vi "RunTest.vi"(8 "error in (no error)":errorcluster, 11 "Prueba08 in":refnum<class "Prueba08.lvclass">) -> (0 "error out":errorcluster, 2 "resultado":string, 3 "Prueba08 out":refnum<class "Prueba08.lvclass">)   [LabVIEW 2019, in "Prueba08.lvclass"]
uses:
  Prueba08.lvclass
  Prueba04/Control/Slide.ctl
  MessageP08.ctl
  Controles/EstadosP08.ctl
  Prueba08.lvclass/Prueba08.ctl
  ClusterGEN.ctl
  <vilib>/Utility/error.llb/DialogType.ctl
  QMH/Message Queue/Enqueue Message (Single).vi
  <vilib>/Utility/error.llb/Error Cluster From Error Code.vi
  <vilib>/ErrorRing/Error Ring.xnode
  <vilib>/Utility/miscctls.llb/LVRowAndColumnTypeDef.ctl
  Prueba/Prueba.lvclass
  Prueba04/Prueba04.lvclass
  QMH/User Event - Stop/User Event - Stop.lvlib
  QMH/Message Queue/Message Queue.lvlib
panel:
  out "Leq":bool
  out "data":string
  out "fila_tabla":i32
  out "ms":dbl
  out "ms":string[](array[string])
  out "max value":dbl
  out "tablaTipoPondTemp":string[](array[string])
  out "tablaNivelMaxRef":string[](array[string])
  out "Pict Ring 2":u16(ring)
  out "Pict Ring 3":u16(ring)
  out "cumple_no_cumple":bool
  out "Vref":dbl
  in  "Tab":enum32{"Page 1", "Page 2"}(tab)
  out "NivelRMSensayo":dbl=95.0
  out "frecuencia1":dbl=140.0
  out "rangoRef":string
  in  "guardar_Vref":bool
  in  "generar1":bool
  in  "AjusteAmp":T1=50.0 caption="Ajuste de amplitud [mV]" scale=0.0..5000.0
  out "voltaje1":dbl format="%.1f"
  out "frecuencia1":dbl format="%.1f"
  in  "seguir":bool
  in  "guardarParamLEQ":bool caption="PruebaSup"
  in  "Tm":i32=60 min=60
  in  "N":i32=1 min=1 max=9
  in  "TablaTempotal":string[][](table)
  in  "cb_ponderacionTemp":string(combo)="0"
  in  "genera2":bool caption="PruebaSup"
  out "Tabla":string[][](table)
  in  "salir":bool
  out "cumple":bool
  out "no_cumple":bool
  out "voltaje2":dbl format="%#.1f"
  out "frecuencia2":dbl format="%#.1f"
  # "Elección Señal de Referencia\nsegún marca y modelo de sonómetro"
  # "Nivel RMS para Ensayo"
  # "Rango Referencia"
  # "Frecuencia"
  # "Monitoreo"
  # "Frecuencia"
  # "Hz"
  # "Voltaje"
  # "mV"
  # "8. Respuesta a trenes de ondas. IEC 61672-3: 2006 Cláusula 16"
  # "Tabla Resultados"
  # "Ingrese mediciones\naquí"
  # "Ingrese parámetros"
  # "Seleccione Tone Burst"
  # "N"
  # "Tm"
  # "Solo el máximo valor se \nregistrará en la tabla de Resultados"
  # "Cumple"
  # "No Cumple"
  # "8. Respuesta a trenes de ondas. IEC 61672-3: 2006 Cláusula 16"
  # "Monitoreo"
  # "Nivel RMS para Ensayo"
  # "dB"
  # "Voltaje"
  # "mV"
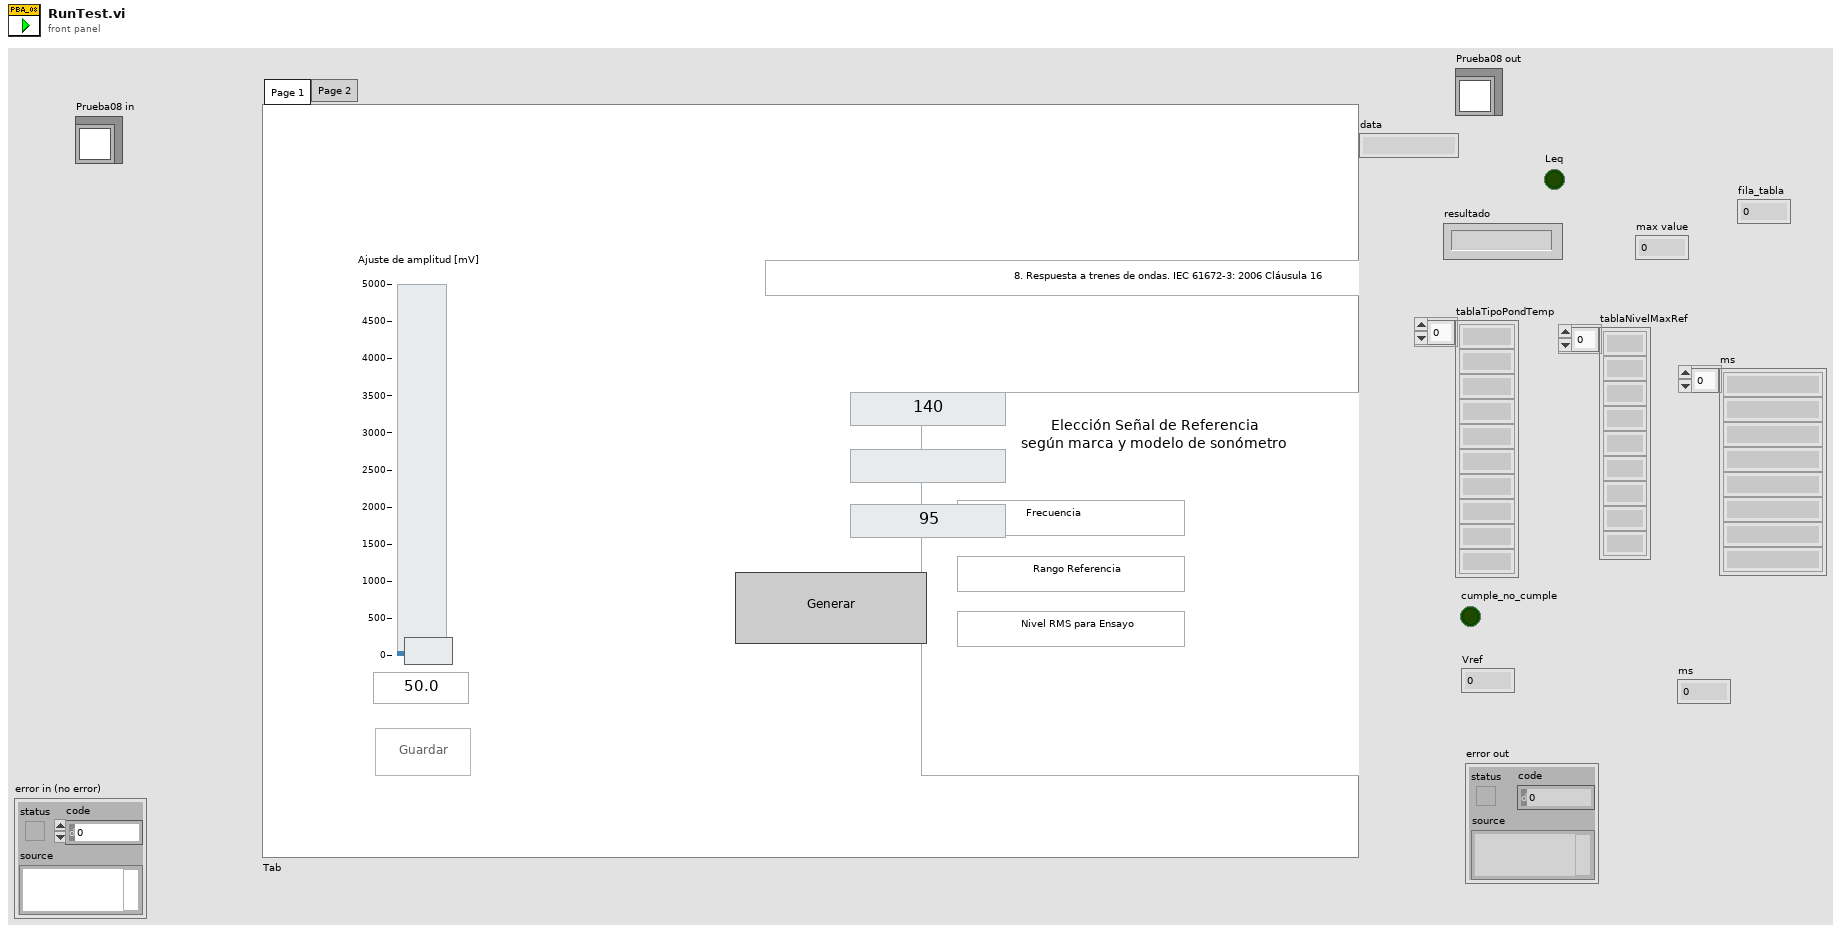
[diagram p1: front panel]
types:
  T1 = typedef "Prueba04.lvclass/Slide.ctl" = dbl
  T2 = typedef "LVRowAndColumnTypeDef.ctl" = cluster{"Row":i32, "Column":i32}
  T3 = typedef "Message Queue.lvlib/All Message Queues.ctl" = cluster{"MHL":refnum<queue>, "Inst_CNT90":refnum<queue>, "Inst_DS360":refnum<queue>, "Inst_Keithley2002":refnum<queue>, "Inst_DAQ":refnum<queue>, "BD":refnum<queue>, "Pistofono":refnum<queue>, "Nexus":refnum<queue>}
  T4 = enum32{"Page 1", "Page 2", "Page 3", "Page 4", "Page 5", "Page 6", "Page 7"}
  T5 = typedef "Prueba08.lvclass/ClusterGEN.ctl" = cluster{"frec":dbl, "amp":dbl, "ms_burst":dbl}
  T6 = enum8{"Enabled", "Disabled", "Disabled and Grayed Out"}
  T7 = cluster{"ControlName":string, "ControlReference":refnum<vi>}[]
  T8 = typedef "Prueba08.lvclass/MessageP08.ctl" = cluster{"Estados":T9, "Data":variant}
  T9 = typedef "Prueba08.lvclass/EstadosP08.ctl" = enum16{"Error", "DetieneInstrumentos", "InicializarInstrumentos", "inicio", "configuraTabla", "FrecAmp1", "FrecAmp2", "nivelMaxRef", "iniciarGEN", "iniciarGEN_burst", "detenerGEN", "llenaTablaTemporal", "guardaVref", "monitoreo", "ingresaMediciones", "guardaMediciones", "cumplimiento", "listo_evaluar", "evaluar", "LeerArchivoConfiguracion", "final", "salir"}
  T10 = typedef "DialogType.ctl" = u16
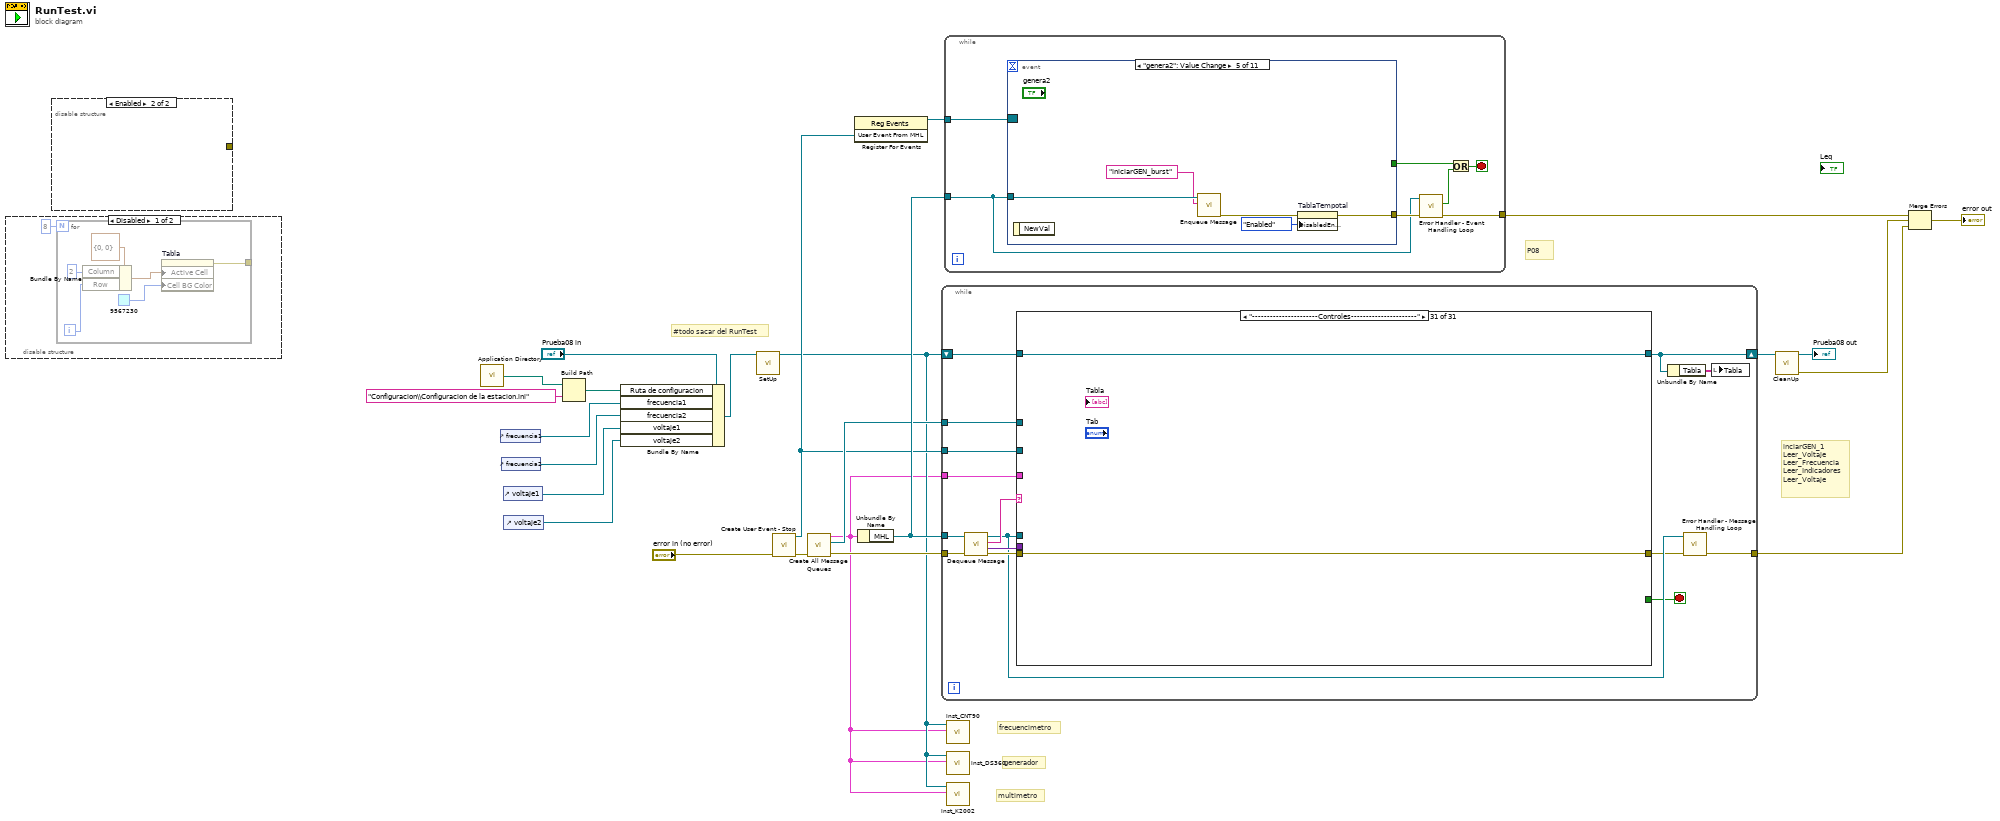
[diagram p0: block diagram]
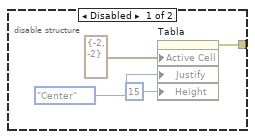
[diagram p3: hidden frame]
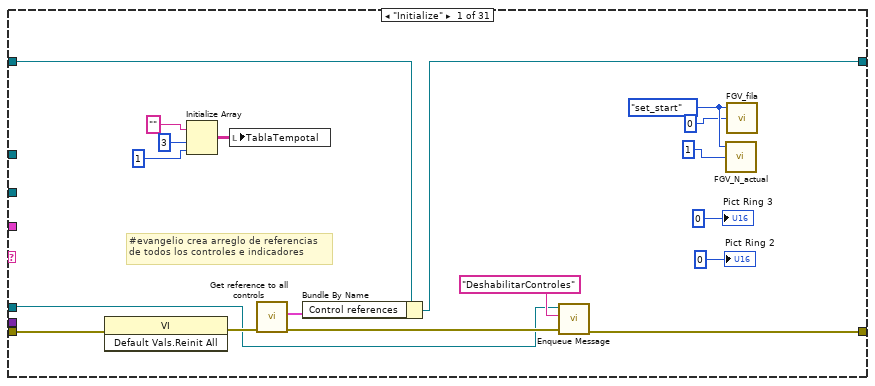
[diagram p4: hidden frame]
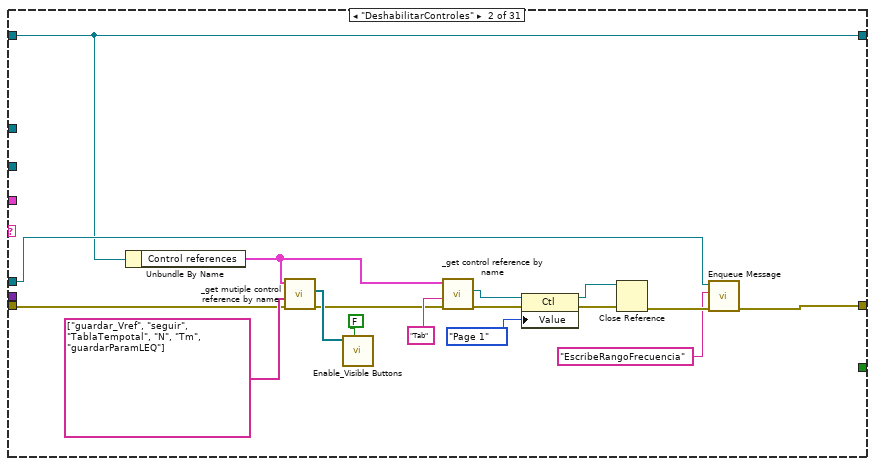
[diagram p5: hidden frame]
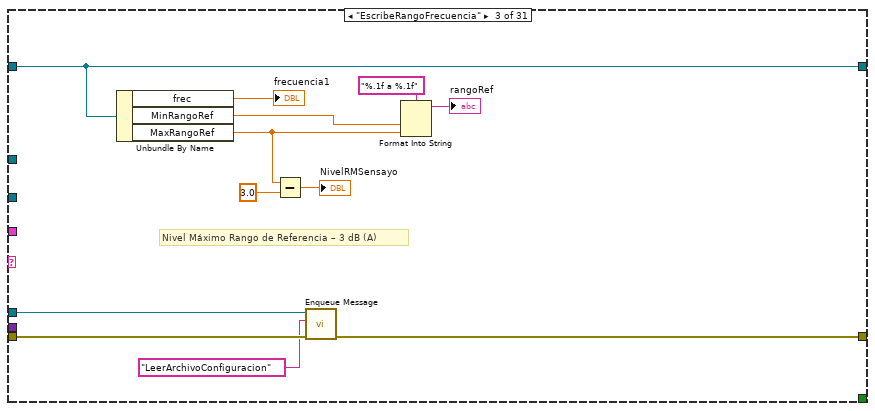
[diagram p6: hidden frame]
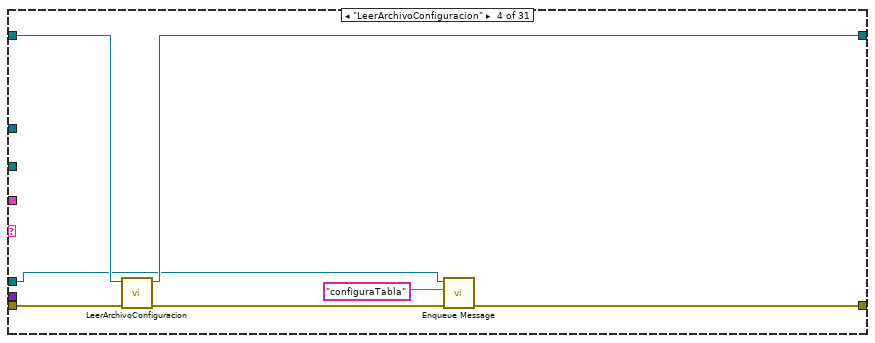
[diagram p7: hidden frame]
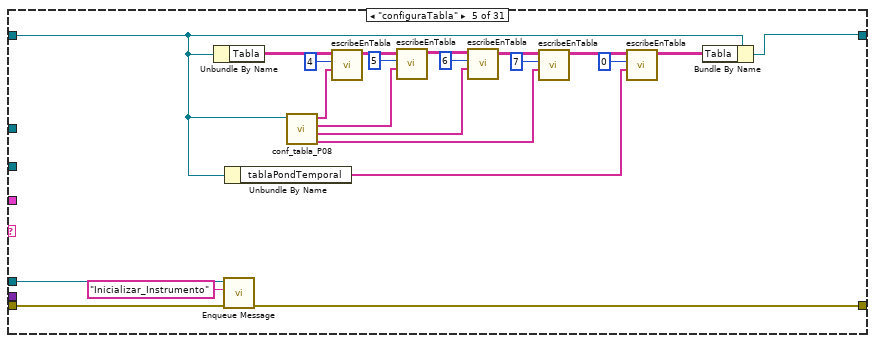
[diagram p8: hidden frame]
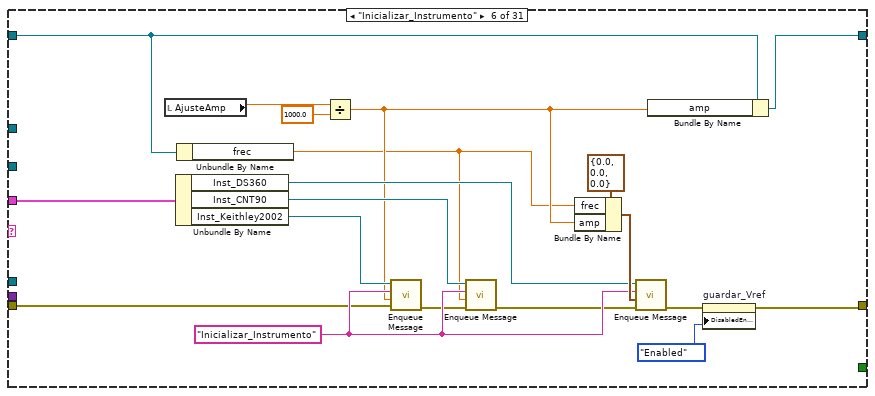
[diagram p9: hidden frame]
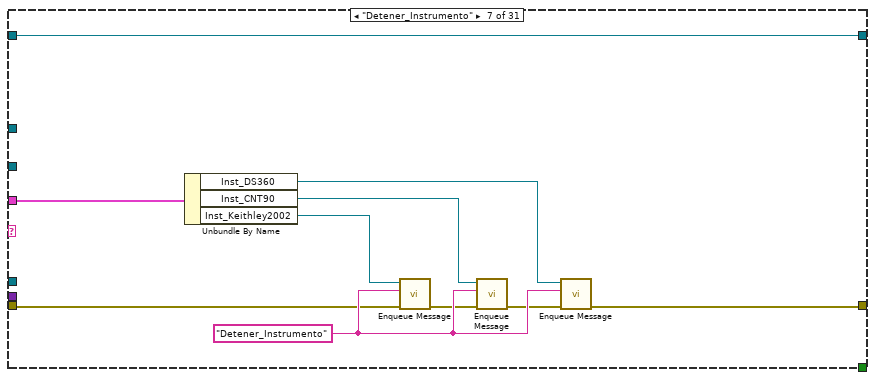
[diagram p10: hidden frame]
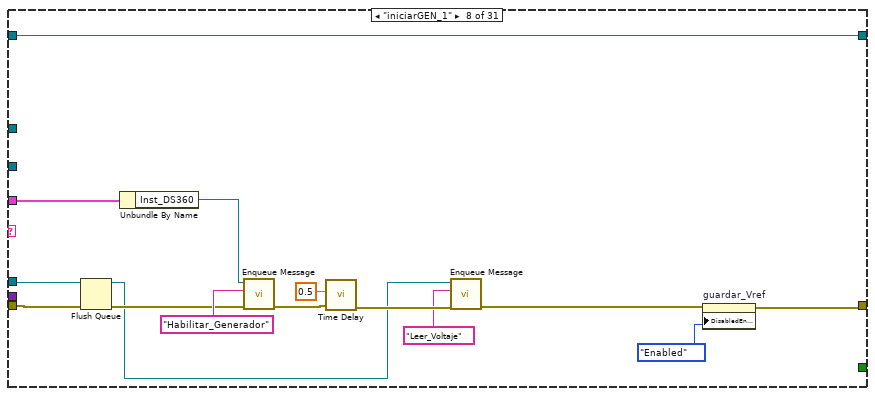
[diagram p11: hidden frame]
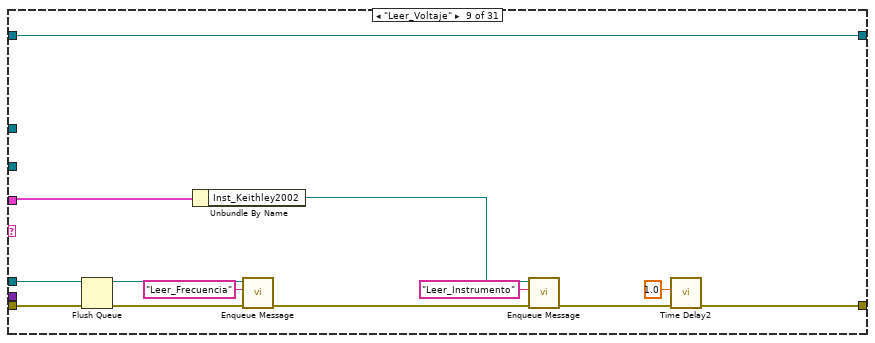
[diagram p12: hidden frame]
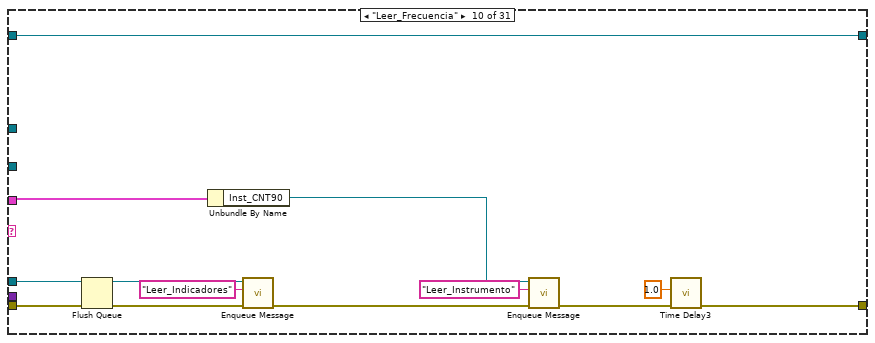
[diagram p13: hidden frame]
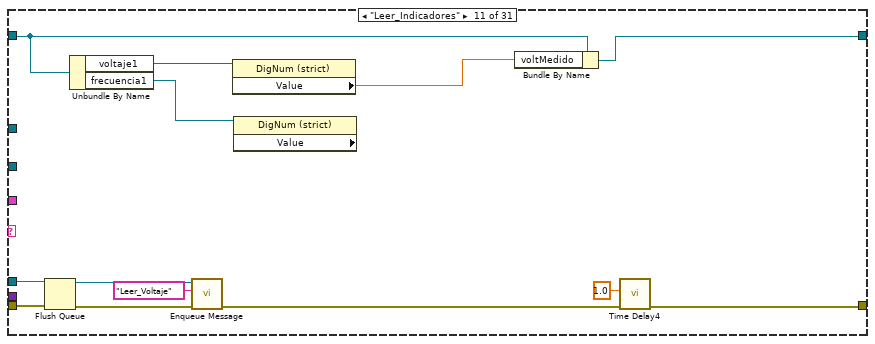
[diagram p14: hidden frame]
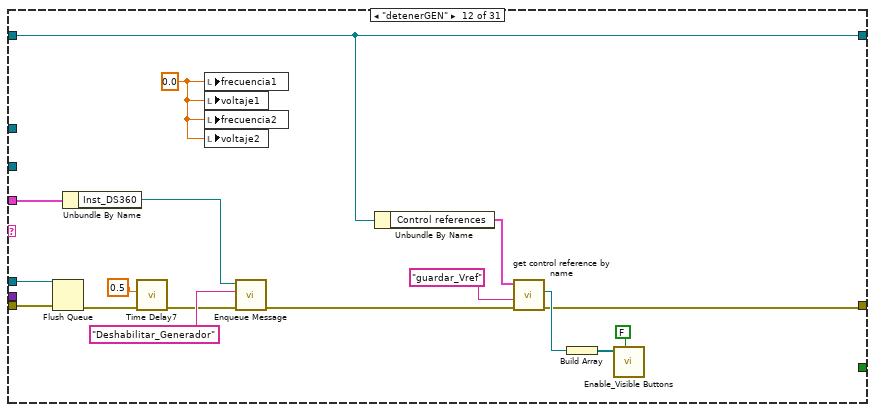
[diagram p15: hidden frame]
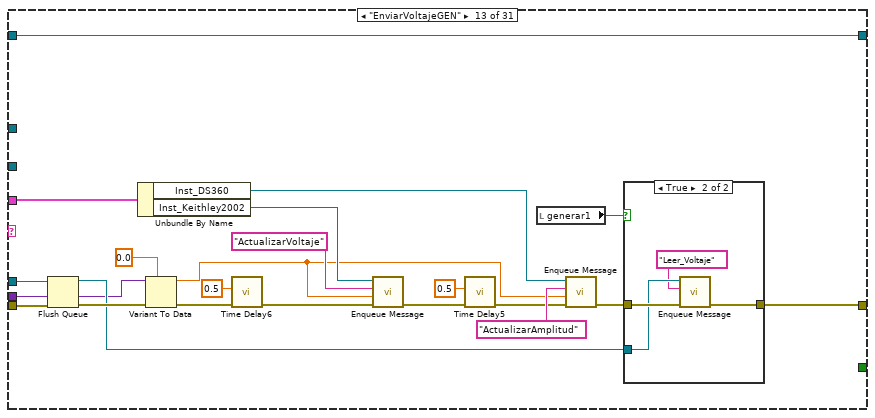
[diagram p16: hidden frame]
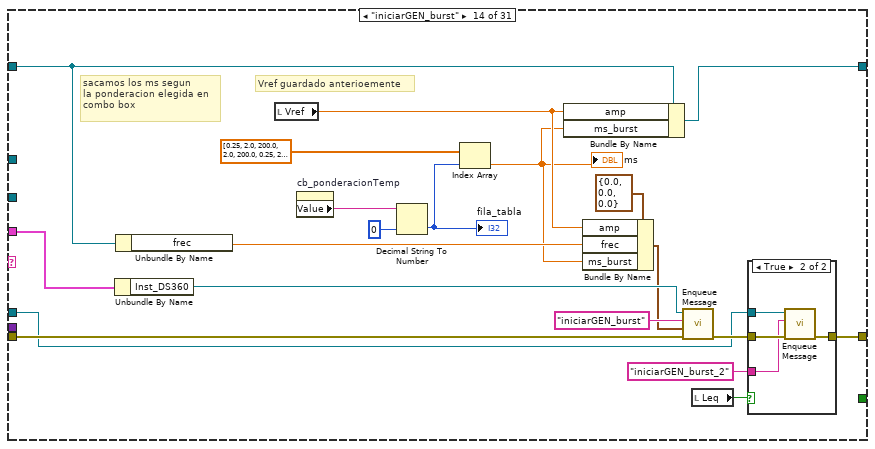
[diagram p18: hidden frame]
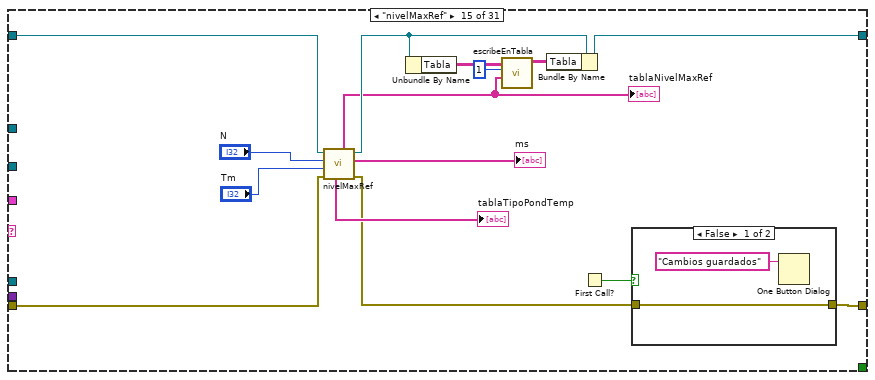
[diagram p20: hidden frame]
diagram:
  # "inciarGEN_1\nLeer_Voltaje\nLeer_Frecuencia\nLeer_Indicadores\nLeer_Voltaje"
  # "P08"
  # "multimetro"
  # "generador"
  # "frecuencimetro"
  # "#todo sacar del RunTest"
  n1 = disable-structure shown="Disabled" {
    frame Disabled {
      n2 = for {
        N: 8 -> [_]
        tunnel: [w27] -> _
        i -> [w26]
        n3 = Bundle By Name(cluster=T2 {"Row"=0, "Column"=0} ("Active Cell:Active Cell"), "Column"=2, "Row"=w26) -> (w29:T2)
        n4 = property on="Tabla" class="Tbl (strict)"("Active Cell"=w29, "Cell BG Color"=u32 9567230) -> (error out=w27:errorcluster)  [unwired: 2 in, 1 out]
      }
    }
    frame Enabled {
    }
  }
  n5 = disable-structure shown="Enabled" {
    disable-tunnel: [w34 _] -> _
    frame Disabled {
      n6 = property on="Tabla" class="Tbl (strict)"("Active Cell"=T2 {"Row"=-2, "Column"=-2} ("Active Cell:Active Cell"), "Justify"=enum16{"Left", "Center", "Right"}."Center" ("Active Cell:Cell Justification"), "Height"=u32 15 ("Active Cell:Cell Font:Size")) -> (error out=w34:errorcluster)  [unwired: 2 in, 1 out]
    }
    frame Enabled {
    }
  }
  n7 = call <vilib>:"Application Directory.vi"() -> ("Application Directory"=w19:path)
  n8 = control-ref of="frecuencia1"() -> (w8:refnum<vi>)
  n9 = control-ref of="frecuencia2"() -> (w7:refnum<vi>)
  n10 = control-ref of="voltaje1"() -> (w6:refnum<vi>)
  n11 = control-ref of="voltaje2"() -> (w5:refnum<vi>)
  n12 = Build Path(base path=w19, name or relative path="Configuracion\\Configuracion de la estacion.ini") -> (appended path=w18:path)
  n13 = Bundle By Name(cluster="Prueba08 in", "Ruta de configuracion"=w18, "frecuencia1"=w8, "frecuencia2"=w7, "voltaje1"=w6, "voltaje2"=w5) -> (w21:refnum<class "Prueba08.lvclass">)
  n14 = call-dynamic "SetUp.vi"("Prueba08 in"=w21) -> ("Prueba08 out"=w10:refnum<class "Prueba08.lvclass">)  [unwired: 9 in, 1 out]
  n15 = call "Create User Event - Stop.vi"("error in (no error)"="error in (no error)") -> ("error out"=w17:errorcluster, "User Event From MHL"=w12:refnum<user-event>)  [unwired: 9 in]
  n16 = call "Create All Message Queues.vi"("error in (no error)"=w17) -> ("error out"=w14:errorcluster, "PL Queues Array"=w13:refnum<queue>[], "All Message Queues out"=w9:T3)  [unwired: 8 in]
  n17 = register-events(w12) -> (reference out=w11:refnum<event-registration>)  [unwired: 2 in, 1 out]
  n18 = Unbundle By Name(w9) -> ("MHL"=w15:refnum<queue>)
  n19 = while {
    tunnel: w15 -> [w47]
    tunnel: w14 -> [w46]
    tunnel: [w40] -> w2
    shift-right: [w48] -> w4
    shift-left: w10 -> [w49]
    tunnel: w9 -> [w39]
    tunnel: w13 -> [w38]
    tunnel: w12 -> [w37]
    stop <- w36 stop-if-true
    n20 = call "Dequeue Message.vi"("error in (no error)"=w46, "Message Queue"=w47) -> ("error out"=w45:errorcluster, "Message Data"=w44:variant, "Message"=w43:string, "dup Message Queue"=w42:refnum<queue>)  [unwired: 6 in]
    n21 = case shown="\"----------------------Controles----------------------\"" w43 {
      selector: w43 -> [_ _ _ _ _ _ _ _ _ _ _ _ _ _ _ _ _ _ _ _ _ _ _ _ _ _ _ w474 _ w504 _]
      tunnel: w44 -> [_ _ _ _ _ _ _ _ _ _ _ _ w229 _ _ w305 w333 _ _ _ _ _ _ w434 w445 _ w468 _ _ _ _]
      tunnel: w45 -> [w64 w72 w89 w104 w120 w133 w148 w169 w174 w187 w204 w218 w231 w273 w292 w306 w340 w355 w372 w381 w397 w403 w415 w437 w448 w450 w469 w478 w489 _ w513]
      tunnel: [w62 w69 w86 w98 w107 w129 w147 w166 w171 w184 w200 w220 w228 w257 w280 w299 w339 w356 w370 w380 w395 w403 w419 w431 w443 w449 w463 w471 w487 w503 w513] -> w41
      tunnel: w42 -> [w63 w71 w88 w100 w106 _ _ w168 w173 w186 w203 w217 w230 w256 _ _ w337 w353 w369 w379 w396 _ w420 _ _ _ w462 w477 w488 _ _]
      tunnel: [w53 w70 w97 w103 w117 w145 w155 w165 w183 w196 w201 w216 w248 w272 w287 w302 w334 w364 w368 w376 w393 w404 w422 w435 w446 w453 w470 w473 w494 w505 w514] -> w48
      tunnel: w49 -> [w54 w70 w97 w102 w109 w128 w155 w165 w183 w196 w202 w216 w248 w261 w293 w302 w334 w365 w367 w376 w393 w404 w422 w436 w447 w453 w470 w473 w494 w505 w514]
      tunnel: w39 -> [_ _ _ _ _ w132 w146 w167 w172 w185 _ w219 w232 w267 _ _ _ _ _ _ _ _ _ _ _ _ _ _ _ _ _]
      tunnel: w38 -> [_ _ _ _ _ _ _ _ _ _ _ _ _ _ _ _ _ _ _ _ _ _ _ _ _ _ _ w476 _ _ _]
      tunnel: w37 -> [_ _ _ _ _ _ _ _ _ _ _ _ _ _ _ _ _ _ _ _ _ _ _ _ _ _ _ w475 _ _ _]
      tunnel: [_ _ _ _ _ _ _ _ _ _ _ _ _ _ _ _ _ _ _ _ _ _ _ _ _ _ _ w472 _ _ _] -> w36
      frame "Initialize" {
        w56 = enum16{"increment", "set_start", "get"}."set_start" ("action")
        # "#evangelio crea arreglo de referencias\nde todos los controles e indicadores"
        n22 = invoke class="VI" method="Default Vals.Reinit All"(error in=w64) -> (error out=w67:errorcluster)  [unwired: 2 in, 2 out]
        n23 = Initialize Array("", 3 ("dimension size"), 1 ("dimension size")) -> (w61:string[][])
        n24 = local write "TablaTempotal"(w61) -> ()
        n25 = call "Get reference to all controls.vi"("error in (no error)"=w67) -> ("error out"=w65:errorcluster, "Control references"=w66:T7)  [unwired: 5 in]
        n26 = Bundle By Name(cluster=w54, "Control references"=w66) -> (w53:refnum<class "Prueba08.lvclass">)
        n27 = call-poly "Enqueue Message.vi"("error in (no error)"=w65, "Message"="DeshabilitarControles", "Message Queue"=w63) -> ("error out"=w62:errorcluster)  [unwired: 7 in, 1 out]
        n28 = call "FGV_N_actual.vi"("N_actual in"=1 ("fila_inicial"), "action"=w56) -> ()  [unwired: 2 in, 2 out]
        n29 = call "FGV_fila.vi"("fila_inicial"=0, "action"=w56) -> ()  [unwired: 2 in, 2 out]
        "Pict Ring 2" <- u16 0 ("Pict Ring 2")
        "Pict Ring 3" <- u16 0 ("Pict Ring 3")
      }
      frame "DeshabilitarControles" {
        n30 = Unbundle By Name(w70) -> ("Control references"=w81:T7)
        n31 = call "_get mutiple control reference by name.vi"("error in (no error)"=w72, "Control names"=string[] ["guardar_Vref", "seguir", "TablaTempotal", "N", "Tm", "guardarParamLEQ"], "Control references"=w81) -> ("error out"=w78:errorcluster, "References"=w79:refnum<vi>[])  [unwired: 3 in]
        n32 = call "Enable_Visible Buttons.vi"("Enable? (T)"=FALSE, "Controls Ref Array"=w79) -> ()  [unwired: 10 in]
        n33 = call "_get control reference by name.vi"("error in (no error)"=w78, "Control name"="Tab" ("Message"), "Control references"=w81) -> ("error out"=w85:errorcluster, "Ctl Refnum"=w83:refnum<vi>)  [unwired: 3 in]
        n34 = property class="Ctl"(reference=w83, error in=w85, "Value"=T4."Page 1" ("Tab_Prueba04")) -> (reference out=w74:refnum<vi>, error out=w76:errorcluster)
        n35 = Close Reference(reference=w74, error in (no error)=w76) -> (error out=w75:errorcluster)
        n36 = call-poly "Enqueue Message.vi"("error in (no error)"=w75, "Message"="EscribeRangoFrecuencia", "Message Queue"=w71) -> ("error out"=w69:errorcluster)  [unwired: 7 in, 1 out]
      }
      frame "EscribeRangoFrecuencia" {
        # "Nivel Máximo Rango de Referencia – 3 dB (A)"
        n37 = Unbundle By Name(w97) -> ("frec"=→"frecuencia1":dbl, "MinRangoRef"=w93:dbl, "MaxRangoRef"=w92:dbl)
        n38 = Subtract(x=w92, y=3.0) -> (x-y=→"NivelRMSensayo":dbl)
        n39 = call-poly "Enqueue Message.vi"("error in (no error)"=w89, "Message"="LeerArchivoConfiguracion", "Message Queue"=w88) -> ("error out"=w86:errorcluster)  [unwired: 7 in, 1 out]
        n40 = Format Into String(format string="%.1f a %.1f", w93, w92) -> (resulting string=→"rangoRef":string)  [unwired: 2 in, 1 out]
      }
      frame "LeerArchivoConfiguracion" {
        n41 = call "LeerArchivoConfiguracion.vi"("error in"=w104, "Prueba31 in"=w102) -> ("error out"=w101:errorcluster, "Prueba31 out"=w103:refnum<class "Prueba08.lvclass">)  [unwired: 8 in]
        n42 = call-poly "Enqueue Message.vi"("error in (no error)"=w101, "Message"="configuraTabla", "Message Queue"=w100) -> ("error out"=w98:errorcluster)  [unwired: 7 in, 1 out]
      }
      frame "configuraTabla" {
        n43 = Unbundle By Name(w109) -> ("Tabla"=w116:string[][])
        n44 = call-poly "Enqueue Message.vi"("error in (no error)"=w120, "Message"="Inicializar_Instrumento", "Message Queue"=w106) -> ("error out"=w107:errorcluster)  [unwired: 7 in, 1 out]
        n45 = Unbundle By Name(w109) -> ("tablaPondTemporal"=w108:string[])
        n46 = call "conf_tabla_P08.vi"("Prueba07 out"=w109) -> ("cumplimiento"=w112:string[], "Tol -"=w113:string[], "Tol +"=w114:string[], "incertidumbre"=w115:string[])  [unwired: 7 in]
        n47 = call "escribeEnTabla.vi"("parametros"=w115, "col"=4, "tabla in"=w116) -> ("tabla out"=w126:string[][])  [unwired: 8 in]
        n48 = call "escribeEnTabla.vi"("parametros"=w114, "col"=5, "tabla in"=w126) -> ("tabla out"=w125:string[][])  [unwired: 8 in]
        n49 = call "escribeEnTabla.vi"("parametros"=w113, "col"=6, "tabla in"=w125) -> ("tabla out"=w121:string[][])  [unwired: 8 in]
        n50 = call "escribeEnTabla.vi"("parametros"=w112, "col"=7, "tabla in"=w121) -> ("tabla out"=w119:string[][])  [unwired: 8 in]
        n51 = call "escribeEnTabla.vi"("parametros"=w108, "col"=0, "tabla in"=w119) -> ("tabla out"=w111:string[][])  [unwired: 8 in]
        n52 = Bundle By Name(cluster=w109, "Tabla"=w111) -> (w117:refnum<class "Prueba08.lvclass">)
      }
      frame "Inicializar_Instrumento" {
        w140 = "Inicializar_Instrumento" ("Message")
        n53 = local read "AjusteAmp"() -> (w144:T1)
        n54 = Unbundle By Name(w132) -> ("Inst_DS360"=w135:refnum<queue>, "Inst_CNT90"=w134:refnum<queue>, "Inst_Keithley2002"=w142:refnum<queue>)
        n55 = Unbundle By Name(w128) -> ("frec"=w127:dbl)
        n56 = Divide(x=w144, y=T1 1000.0) -> (x/y=w130:T1)
        n57 = call-poly "Enqueue Message.vi"("error in (no error)"=w133, "Message Data"=w130, "Message"=w140, "Message Queue"=w142) -> ("error out"=w139:errorcluster)  [unwired: 6 in, 1 out]
        n58 = call-poly "Enqueue Message.vi"("error in (no error)"=w139, "Message Data"=w127, "Message"=w140, "Message Queue"=w134) -> ("error out"=w138:errorcluster)  [unwired: 6 in, 1 out]
        n59 = Bundle By Name(cluster=T5 {"frec"=0.0, "amp"=0.0, "ms_burst"=0.0} ("clusterGEN"), "frec"=w127, "amp"=w130) -> (w141:T5)
        n60 = call-poly "Enqueue Message.vi"("error in (no error)"=w138, "Message Data"=w141, "Message"=w140, "Message Queue"=w135) -> ("error out"=w136:errorcluster)  [unwired: 6 in, 1 out]
        n61 = Bundle By Name(cluster=w128, "amp"=w130) -> (w145:refnum<class "Prueba08.lvclass">)
        n62 = property on="guardar_Vref" class="Bool"(error in=w136, "DisabledEnum"=T6."Enabled" ("Disabled")) -> (error out=w129:errorcluster)  [unwired: 1 in, 1 out]
      }
      frame "Detener_Instrumento" {
        w151 = "Detener_Instrumento" ("Message")
        n63 = Unbundle By Name(w146) -> ("Inst_DS360"=w154:refnum<queue>, "Inst_CNT90"=w153:refnum<queue>, "Inst_Keithley2002"=w152:refnum<queue>)
        n64 = call-poly "Enqueue Message.vi"("error in (no error)"=w148, "Message"=w151, "Message Queue"=w152) -> ("error out"=w150:errorcluster)  [unwired: 7 in, 1 out]
        n65 = call-poly "Enqueue Message.vi"("error in (no error)"=w150, "Message"=w151, "Message Queue"=w153) -> ("error out"=w149:errorcluster)  [unwired: 7 in, 1 out]
        n66 = call-poly "Enqueue Message.vi"("error in (no error)"=w149, "Message"=w151, "Message Queue"=w154) -> ("error out"=w147:errorcluster)  [unwired: 7 in, 1 out]
      }
      frame "iniciarGEN_1" {
        n67 = Flush Queue(queue=w168, error in (no error)=w169) -> (queue out=w156:refnum<queue>, error out=w159:errorcluster)  [unwired: 1 out]
        n68 = Unbundle By Name(w167) -> ("Inst_DS360"=w157:refnum<queue>)
        n69 = call-poly "Enqueue Message.vi"("error in (no error)"=w159, "Message"="Habilitar_Generador", "Message Queue"=w157) -> ("error out"=w162:errorcluster)  [unwired: 7 in, 1 out]
        n70 = call "Time Delay"("error in (no error)"=w162, "Delay Time (s)"=0.5) -> ("error out"=w161:errorcluster)  [unwired: 9 in]
        n71 = call-poly "Enqueue Message.vi"("error in (no error)"=w161, "Message"="Leer_Voltaje", "Message Queue"=w156) -> ("error out"=w158:errorcluster)  [unwired: 7 in, 1 out]
        n72 = property on="guardar_Vref" class="Bool"(error in=w158, "DisabledEnum"=T6."Enabled" ("Disabled")) -> (error out=w166:errorcluster)  [unwired: 1 in, 1 out]
      }
      frame "Leer_Voltaje" {
        n73 = Flush Queue(queue=w173, error in (no error)=w174) -> (queue out=w175:refnum<queue>, error out=w176:errorcluster)  [unwired: 1 out]
        n74 = Unbundle By Name(w172) -> ("Inst_Keithley2002"=w179:refnum<queue>)
        n75 = call-poly "Enqueue Message.vi"("error in (no error)"=w176, "Message"="Leer_Frecuencia", "Message Queue"=w175) -> ("error out"=w182:errorcluster)  [unwired: 7 in, 1 out]
        n76 = call-poly "Enqueue Message.vi"("error in (no error)"=w182, "Message"="Leer_Instrumento", "Message Queue"=w179) -> ("error out"=w180:errorcluster)  [unwired: 7 in, 1 out]
        n77 = call "Time Delay2"("error in (no error)"=w180, "Delay Time (s)"=1.0) -> ("error out"=w171:errorcluster)  [unwired: 9 in]
      }
      frame "Leer_Frecuencia" {
        n78 = Flush Queue(queue=w186, error in (no error)=w187) -> (queue out=w188:refnum<queue>, error out=w189:errorcluster)  [unwired: 1 out]
        n79 = Unbundle By Name(w185) -> ("Inst_CNT90"=w192:refnum<queue>)
        n80 = call-poly "Enqueue Message.vi"("error in (no error)"=w189, "Message"="Leer_Indicadores", "Message Queue"=w188) -> ("error out"=w195:errorcluster)  [unwired: 7 in, 1 out]
        n81 = call-poly "Enqueue Message.vi"("error in (no error)"=w195, "Message"="Leer_Instrumento", "Message Queue"=w192) -> ("error out"=w193:errorcluster)  [unwired: 7 in, 1 out]
        n82 = call "Time Delay3"("error in (no error)"=w193, "Delay Time (s)"=1.0) -> ("error out"=w184:errorcluster)  [unwired: 9 in]
      }
      frame "Leer_Indicadores" {
        n83 = Flush Queue(queue=w203, error in (no error)=w204) -> (queue out=w205:refnum<queue>, error out=w206:errorcluster)  [unwired: 1 out]
        n84 = Unbundle By Name(w202) -> ("voltaje1"=w199:refnum<vi>, "frecuencia1"=w198:refnum<vi>)
        n85 = call-poly "Enqueue Message.vi"("error in (no error)"=w206, "Message"="Leer_Voltaje", "Message Queue"=w205) -> ("error out"=w209:errorcluster)  [unwired: 7 in, 1 out]
        n86 = property class="DigNum (strict)"(reference=w199) -> ("Value"=w197:dbl)  [unwired: 1 in, 2 out]
        n87 = property class="DigNum (strict)" props=["Value"](reference=w198) -> ()  [unwired: 1 in, 3 out]
        n88 = Bundle By Name(cluster=w202, "voltMedido"=w197) -> (w201:refnum<class "Prueba08.lvclass">)
        n89 = call "Time Delay4"("error in (no error)"=w209, "Delay Time (s)"=1.0) -> ("error out"=w200:errorcluster)  [unwired: 9 in]
      }
      frame "detenerGEN" {
        w215 = 0.0 ("frecuencia1")
        n90 = Flush Queue(queue=w217, error in (no error)=w218) -> (error out=w212:errorcluster)  [unwired: 2 out]
        n91 = Unbundle By Name(w219) -> ("Inst_DS360"=w226:refnum<queue>)
        n92 = call "Time Delay7"("error in (no error)"=w212, "Delay Time (s)"=0.5) -> ("error out"=w211:errorcluster)  [unwired: 9 in]
        n93 = local write "frecuencia1"(w215) -> ()
        n94 = local write "voltaje1"(w215) -> ()
        n95 = local write "frecuencia2"(w215) -> ()
        n96 = local write "voltaje2"(w215) -> ()
        n97 = call-poly "Enqueue Message.vi"("error in (no error)"=w211, "Message"="Deshabilitar_Generador", "Message Queue"=w226) -> ("error out"=w210:errorcluster)  [unwired: 7 in, 1 out]
        n98 = Unbundle By Name(w216) -> ("Control references"=w221:T7)
        n99 = call-poly "get control reference by name.vi"("error in (no error)"=w210, "Control name"="guardar_Vref" ("String"), "Control references"=w221) -> ("error out"=w220:errorcluster, "Ctl Refnum"=w223:refnum<vi>)  [unwired: 3 in]
        n100 = Build Array(w223) -> (w222:refnum<vi>[])
        n101 = call "Enable_Visible Buttons.vi"("Enable? (T)"=FALSE, "Controls Ref Array"=w222) -> ()  [unwired: 10 in]
      }
      frame "EnviarVoltajeGEN" {
        n102 = Flush Queue(queue=w230, error in (no error)=w231) -> (queue out=w235:refnum<queue>, error out=w238:errorcluster)  [unwired: 1 out]
        n103 = Unbundle By Name(w232) -> ("Inst_DS360"=w242:refnum<queue>, "Inst_Keithley2002"=w247:refnum<queue>)
        n104 = Variant To Data(error in=w238, type=0.0, Variant=w229) -> (data=w240:dbl, error out=w245:errorcluster)
        n105 = call "Time Delay6"("error in (no error)"=w245, "Delay Time (s)"=0.5) -> ("error out"=w234:errorcluster)  [unwired: 9 in]
        n106 = call-poly "Enqueue Message.vi"("error in (no error)"=w234, "Message Data"=w240, "Message"="ActualizarVoltaje", "Message Queue"=w247) -> ("error out"=w243:errorcluster)  [unwired: 6 in, 1 out]
        n107 = call "Time Delay5"("error in (no error)"=w243, "Delay Time (s)"=0.5) -> ("error out"=w237:errorcluster)  [unwired: 9 in]
        n108 = local read "generar1"() -> (w227:bool)
        n109 = call-poly "Enqueue Message.vi"("error in (no error)"=w237, "Message Data"=w240, "Message"="ActualizarAmplitud", "Message Queue"=w242) -> ("error out"=w239:errorcluster)  [unwired: 6 in, 1 out]
        n110 = case shown="True" w227 {
          tunnel: w239 -> [w249 w253]
          tunnel: [w249 w252] -> w228
          tunnel: w235 -> [_ w251]
          frame False {
          }
          frame True {
            n111 = call-poly "Enqueue Message.vi"("error in (no error)"=w253, "Message"="Leer_Voltaje", "Message Queue"=w251) -> ("error out"=w252:errorcluster)  [unwired: 7 in, 1 out]
          }
        }
      }
      frame "iniciarGEN_burst" {
        # "sacamos los ms segun\nla ponderacion elegida en\ncombo box"
        # "Vref guardado anterioemente"
        n112 = Unbundle By Name(w267) -> ("Inst_DS360"=w266:refnum<queue>)
        n113 = Unbundle By Name(w261) -> ("frec"=w260:dbl)
        n114 = local read "Vref"() -> (w262:dbl)
        n115 = property on="cb_ponderacionTemp" class="CmbBox"() -> ("Value"=w270:string)  [unwired: 2 in, 2 out]
        n116 = Decimal String To Number(string=w270, default (0L)=0 ("default (0 I32)")) -> (number=w268:i32)  [unwired: 1 in, 1 out]
        "fila_tabla" <- w268
        n117 = Index Array(array=dbl[] [0.25, 2.0, 200.0, 2.0, 200.0, 0.25, 2.0, 200.0], index=w268) -> (element=w259:dbl)
        "ms" <- w259
        n118 = Bundle By Name(cluster=w261, "amp"=w262, "ms_burst"=w259) -> (w272:refnum<class "Prueba08.lvclass">)
        n119 = Bundle By Name(cluster=T5 {"frec"=0.0, "amp"=0.0, "ms_burst"=0.0} ("clusterGEN"), "amp"=w262, "frec"=w260, "ms_burst"=w259) -> (w263:T5)
        n120 = call-poly "Enqueue Message.vi"("error in (no error)"=w273, "Message Data"=w263, "Message"="iniciarGEN_burst", "Message Queue"=w266) -> ("error out"=w258:errorcluster)  [unwired: 6 in, 1 out]
        n121 = local read "Leq"() -> (w255:bool)
        n122 = case shown="True" w255 {
          tunnel: w258 -> [w274 w278]
          tunnel: [w274 w277] -> w257
          tunnel: w256 -> [_ w276]
          tunnel: "iniciarGEN_burst_2" ("Message") -> [_ w275]
          frame False {
          }
          frame True {
            n123 = call-poly "Enqueue Message.vi"("error in (no error)"=w278, "Message"=w275, "Message Queue"=w276) -> ("error out"=w277:errorcluster)  [unwired: 7 in, 1 out]
          }
        }
      }
      frame "nivelMaxRef" {
        n124 = call "nivelMaxRef.vi"("error in (no error)"=w292, "Tm"="Tm", "N"="N", "Prueba08 in"=w293) -> ("error out"=w281:errorcluster, "ms"=→"ms":string[], "Prueba08 out"=w291:refnum<class "Prueba08.lvclass">, "tablaNivelMaxRef"=w288:string[], "tablaTipoPondTemp"=→"tablaTipoPondTemp":string[])  [unwired: 2 in, 1 out]
        "tablaNivelMaxRef" <- w288
        n125 = Unbundle By Name(w291) -> ("Tabla"=w290:string[][])
        n126 = call "escribeEnTabla.vi"("parametros"=w288, "col"=1, "tabla in"=w290) -> ("tabla out"=w286:string[][])  [unwired: 8 in]
        n127 = Bundle By Name(cluster=w291, "Tabla"=w286) -> (w287:refnum<class "Prueba08.lvclass">)
        n128 = First Call?() -> (First Call?: T/F=w279:bool)
        n129 = case shown="False" w279 {
          tunnel: w281 -> [w294 w296]
          tunnel: [w294 w296] -> w280
          frame False {
            n130 = One Button Dialog(message="Cambios guardados") -> ()  [unwired: 1 in, 1 out]
          }
          frame True {
          }
        }
      }
      frame "TipoPonderacionTemporal" {
        n131 = Variant To Data(error in=w306, type="", Variant=w305) -> (data=w303:string, error out=w300:errorcluster)
        "data" <- w303
        n132 = Unbundle By Name(w302) -> ("Control references"=w301:T7)
        n133 = case shown="\"5\", \"6\", \"7\"" w303 {
          tunnel: w301 -> [w310 w317]
          tunnel: w300 -> [w309 w316]
          tunnel: [w311 w318] -> w299
          tunnel: string[] ["N", "Tm", "guardarParamLEQ"] ("String") -> [w308 w315]
          tunnel: [TRUE FALSE] -> w297
          frame "5", "6", "7" {
            # "Opcion Leq"
            n134 = call-poly "get control reference by name.vi"("error in (no error)"=w309, "Control names"=w308, "Control references"=w310) -> ("error out"=w311:errorcluster, "References"=w312:refnum<vi>[])  [unwired: 3 in]
            n135 = call "Enable_Visible Buttons.vi"("Enable? (T)"=TRUE, "Controls Ref Array"=w312) -> ()  [unwired: 10 in]
          }
          frame Default {
            # "No es Leq"
            n136 = call-poly "get control reference by name.vi"("error in (no error)"=w316, "Control names"=w315, "Control references"=w317) -> ("error out"=w318:errorcluster, "References"=w319:refnum<vi>[])  [unwired: 3 in]
            n137 = call "Enable_Visible Buttons.vi"("Enable? (T)"=FALSE, "Controls Ref Array"=w319) -> ()  [unwired: 10 in]
          }
        }
        n138 = local write "Leq"(w297) -> ()
      }
      frame "llenaTablaTemporal" {
        n139 = Flush Queue(queue=w337, error in (no error)=w340) -> (queue out=w336:refnum<queue>, error out=w338:errorcluster)  [unwired: 1 out]
        n140 = Variant To Data(error in=w338, type=string[][] [] ("NewVal"), Variant=w333) -> (data=w331:string[][], error out=w330:errorcluster)
        n141 = control-ref of="TablaTempotal"() -> (w332:refnum<vi>)
        n142 = call "llenaTablaTemporal.vi"("Tbl Refnum"=w332, "New Value"=w331, "error out"=w330) -> ("max value"=w321:dbl, "error in (no error)"=w329:errorcluster)  [unwired: 6 in]
        "max value" <- w321
        n143 = call "FGV_fila.vi"("error in (no error)"=w329, "action"=enum16{"increment", "set_start", "get"}."increment") -> ("error out"=w328:errorcluster)  [unwired: 2 in, 1 out]
        n144 = call "FGV_fila.vi"("error in (no error)"=w328, "action"=enum16{"increment", "set_start", "get"}."get") -> ("error out"=w326:errorcluster, "fila out"=w324:i32)  [unwired: 2 in]
        n145 = Greater?(x=w324, y=2) -> (0:w322:bool)
        n146 = case shown="True" w322 {
          tunnel: [w341 w350] -> w339
          tunnel: w336 -> [_ w349]
          tunnel: w326 -> [w341 w348]
          tunnel: w321 -> [_ w344]
          frame False {
          }
          frame True {
            n147 = Format Into String(format string="Se ingresará el \\n%.1f a la Tabla" ("message"), w344) -> (resulting string=w343:string)  [unwired: 2 in, 1 out]
            n148 = call "FGV_fila.vi"("fila_inicial"=0, "action"=enum16{"increment", "set_start", "get"}."set_start") -> ()  [unwired: 2 in, 2 out]
            n149 = call-poly "Enqueue Message.vi"("error in (no error)"=w348, "Message"="ingresaMediciones", "Message Queue"=w349) -> ("error out"=w350:errorcluster)  [unwired: 7 in, 1 out]
            n150 = One Button Dialog(message=w343) -> ()  [unwired: 1 in, 1 out]
          }
        }
      }
      frame "ingresaMediciones" {
        (unwired) T8 {"Estados"=enum."cumplimiento", "Data"=variant} ("element")
        # "maximo valor\nencontrado"
        n151 = Flush Queue(queue=w353, error in (no error)=w355) -> (queue out=w352:refnum<queue>, error out=w354:errorcluster)  [unwired: 1 out]
        n152 = property on="TablaTempotal" class="Tbl (strict)"(error in=w354, "Value"=string[][] [] ("TablaTempotal")) -> (error out=w360:errorcluster)  [unwired: 1 in, 1 out]
        n153 = property on="TablaTempotal" class="Tbl (strict)"(error in=w360, "DisabledEnum"=T6."Disabled and Grayed Out" ("Disabled")) -> (error out=w359:errorcluster)  [unwired: 1 in, 1 out]
        n154 = local read "max value"() -> (w363:dbl)
        n155 = local read "fila_tabla"() -> (w362:i32)
        n156 = call "ingresaMediciones.vi"("error in (no error)"=w359, "fila tabla"=w362, "max value"=w363, "Prueba08 in"=w365) -> ("error out"=w357:errorcluster, "Prueba08 out"=w364:refnum<class "Prueba08.lvclass">)  [unwired: 6 in]
        n157 = call-poly "Enqueue Message.vi"("error in (no error)"=w357, "Message"="cumplimiento", "Message Queue"=w352) -> ("error out"=w356:errorcluster)  [unwired: 7 in, 1 out]
      }
      frame "cumplimiento" {
        n158 = call "cumplimiento.vi"("error in (no error)"=w372, "Prueba08 in"=w367) -> ("error out"=w371:errorcluster, "Prueba08 out"=w368:refnum<class "Prueba08.lvclass">)  [unwired: 8 in]
        n159 = call-poly "Enqueue Message.vi"("error in (no error)"=w371, "Message"="listo_evaluar", "Message Queue"=w369) -> ("error out"=w370:errorcluster)  [unwired: 7 in, 1 out]
      }
      frame "listo_evaluar" {
        n160 = Unbundle By Name(w376) -> ("Tabla"=w375:string[][])
        n161 = Index Array(array=w375, index (col)=7 ("disabled index (col)")) -> (element=w374:string[])  [unwired: 1 in]
        n162 = for {
          tunnel: [w389] -> w377 mode=indexing
          tunnel: w374 -> [w387] mode=indexing
          n163 = Not Equal?(x=w387, y="--") -> (x != y?=w389:bool)
        }
        n164 = And Array Elements(Boolean array=w377) -> (logical AND=w373:bool)
        n165 = case shown="True" w373 {
          tunnel: w381 -> [w382 w386]
          tunnel: [w382 w385] -> w380
          tunnel: w379 -> [_ w384]
          frame False {
          }
          frame True {
            (unwired) T8 {"Estados"=enum."evaluar", "Data"=variant} ("MessageP08")
            n166 = call-poly "Enqueue Message.vi"("error in (no error)"=w386, "Message"="evaluar", "Message Queue"=w384) -> ("error out"=w385:errorcluster)  [unwired: 7 in, 1 out]
          }
        }
      }
      frame "evaluar" {
        # "si todos cumplen\nentonces el ensayo\ncumple"
        n167 = Unbundle By Name(w393) -> ("Tabla"=w392:string[][])
        n168 = call-poly "Enqueue Message.vi"("error in (no error)"=w397, "Message"="final", "Message Queue"=w396) -> ("error out"=w395:errorcluster)  [unwired: 7 in, 1 out]
        n169 = Index Array(array=w392, index (col)=7 ("disabled index (col)")) -> (element=w391:string[])  [unwired: 1 in]
        n170 = for {
          tunnel: [w402] -> w399 mode=indexing
          tunnel: w391 -> [w400] mode=indexing
          n171 = Equal?(x=w400, y="Cumple") -> (x = y?=w402:bool)
        }
        n172 = And Array Elements(Boolean array=w399) -> (logical AND=→"cumple_no_cumple":bool)
      }
      frame "final" {
        n173 = local read "cumple_no_cumple"() -> (w405:bool)
        "cumple" <- w405
        n174 = Not(x=w405) -> (.not. x?=→"no_cumple":bool)
        n175 = Select(t="Cumple", s=w405, f="No Cumple") -> (s? t:f=→"resultado":string)
      }
      frame "iniciarGEN_burst_2" {
        n176 = local read "N"() -> (w418:i32)
        n177 = local read "Tm"() -> (w421:i32)
        n178 = call "estadoToneBurst.vi"("error in (no error)"=w415, "Tm"=w421, "N"=w418) -> ("error out"=w413:errorcluster, "Terminar"=w410:bool)  [unwired: 7 in]
        n179 = call "FGV_N_actual.vi"("error in (no error)"=w413, "action"=enum16{"increment", "set_start", "get"}."increment") -> ("error out"=w417:errorcluster, "N_actual out"=w416:i32)  [unwired: 2 in]
        n180 = Greater?(x=w416, y=w418) -> (0:w411:bool)
        n181 = Or(x=w410, y=w411) -> (x .or. y?=w412:bool)
        n182 = case shown="True" w412 {
          tunnel: w420 -> [w426 _]
          tunnel: [w425 w430] -> w419
          tunnel: w417 -> [w424 w430]
          frame False {
            n183 = call-poly "Enqueue Message.vi"("error in (no error)"=w424, "Message"="iniciarGEN_burst", "Message Queue"=w426) -> ("error out"=w425:errorcluster)  [unwired: 7 in, 1 out]
          }
          frame True {
            n184 = One Button Dialog(message="Ingrese las mediciones \nen la Tabla Temporal") -> ()  [unwired: 1 in, 1 out]
            n185 = call "FGV_N_actual.vi"("N_actual in"=1, "action"=enum16{"increment", "set_start", "get"}."set_start") -> ()  [unwired: 2 in, 2 out]
          }
        }
      }
      frame "DatoRecibidoCNT90" {
        n186 = Variant To Data(error in=w437, type=0.0 ("y"), Variant=w434) -> (data=w432:dbl, error out=w431:errorcluster)
        "frecuencia2" <- w432
        "frecuencia1" <- w432
        n187 = Bundle By Name(cluster=w436, "frecMedida"=w432) -> (w435:refnum<class "Prueba08.lvclass">)
      }
      frame "DatoRecibidoK2002" {
        n188 = Variant To Data(error in=w448, type=0.0 ("y"), Variant=w445) -> (data=w439:dbl, error out=w443:errorcluster)
        n189 = Multiply(x=w439, y=1000.0) -> (x*y=w438:dbl)
        "voltaje2" <- w438
        n190 = Multiply(x=w439, y=1000.0) -> (x*y=→"voltaje1":dbl)
        n191 = Bundle By Name(cluster=w447, "voltMedido"=w438) -> (w446:refnum<class "Prueba08.lvclass">)
      }
      frame "guardaVref" {
        n192 = flat-sequence {
          tunnel: [w454] -> w451
          tunnel: w450 -> [w454]
          frame #0 {
            n193 = local read "AjusteAmp"() -> (w457:T1)
            n194 = Divide(x=w457, y=T1 1000.0) -> (x/y=w455:T1)
            "Vref" <- w455
            n195 = Number To Fractional String(number=w455, precision (6)=i16 3) -> (F-format string=w458:string)  [unwired: 2 in]
            n196 = Format Into String(format string="Se guardó Vref = %s volts", w458) -> (resulting string=w461:string)  [unwired: 2 in, 1 out]
            n197 = One Button Dialog(message=w461) -> ()  [unwired: 1 in, 1 out]
          }
        }
        n198 = property on="seguir" class="Bool"(error in=w451, "DisabledEnum"=T6."Enabled" ("Disabled")) -> (error out=w449:errorcluster)  [unwired: 1 in, 1 out]
      }
      frame "Error" {
        w466 = T10 1 items=["no dialog", "OK message", "continue or stop message", "OK message + warnings", "continue/stop + warnings"] ("type of dialog (OK msg:1)")
        n199 = Variant To Data(error in=w469, type=w469, Variant=w468) -> (data=w467:errorcluster, error out=w464:errorcluster)
        n200 = call <vilib>:"Simple Error Handler.vi"("type of dialog (OK msg:1)"=w466, "error in (no error)"=w467) -> ()  [unwired: 3 in, 5 out]
        n201 = call-poly "Enqueue Message.vi"("error in (no error)"=w464, "Message"="Exit", "Message Queue"=w462) -> ("error out"=w463:errorcluster)  [unwired: 7 in, 1 out]
      }
      frame "Exit" {
        w472 = TRUE
        # "#evangelio Manda a cerrar el EHL"
        # "#evangelio Manda a cerrar todos los Loops"
        n202 = Release Queue(queue=w477, error in (no error)=w478) -> (error out=w482:errorcluster)  [unwired: 1 in, 2 out]
        n203 = Unbundle By Name(w473) -> ("Control references"=w483:T7)
        n204 = for {
          tunnel: w476 -> [w486] mode=indexing
          tunnel: w474 -> [w485]
          tunnel: TRUE -> [w484]
          n205 = call-poly "Enqueue Message.vi"("Priority Message? (F)"=w484, "Message"=w485, "Message Queue"=w486) -> ()  [unwired: 7 in, 2 out]
        }
        n206 = call "Close All Ref.vi"("error in (no error)"=w482, "Control references"=w483) -> ("error out"=w480:errorcluster)  [unwired: 9 in]
        n207 = call "Fire User Event - Stop.vi"("error in (no error)"=w480, "Event Data"=w472, "User Event"="Exit EHL", "User Event in"=w475) -> ("error out"=w471:errorcluster)  [unwired: 7 in]
      }
      frame "Confirmar Salida" {
        n208 = Two Button Dialog(message="¿Quieres cerrar la aplicación?", 1:"No" ("T button name (\"OK\")"), 2:"Si" ("T button name (\"OK\")")) -> (T button?=w490:bool)
        n209 = case shown="True" w490 {
          tunnel: w489 -> [w495 w497]
          tunnel: [w495 w502] -> w487
          tunnel: w488 -> [_ w499]
          frame False {
          }
          frame True {
            n210 = call-poly "Enqueue Message.vi"("error in (no error)"=w497, "Message"="Detener_Instrumento", "Message Queue"=w499) -> ("error out"=w496:errorcluster, "dup Message Queue"=w498:refnum<queue>)  [unwired: 7 in]
            n211 = call-poly "Enqueue Message.vi"("error in (no error)"=w496, "Message"="Exit", "Message Queue"=w498) -> ("error out"=w502:errorcluster)  [unwired: 7 in, 1 out]
          }
        }
      }
      frame Default {
        n212 = xnode "Error Ring"("parameter 0"=w504) -> ("error out"=w503:errorcluster)
      }
      frame "----------------------Controles----------------------" {
      }
    }
    n213 = Unbundle By Name(w48) -> ("Tabla"=w50:string[][])
    n214 = call "Error Handler - Message Handling Loop.vi"("error in (no error)"=w41, "Message Queue"=w42) -> ("dup error in"=w40:errorcluster)  [unwired: 8 in, 1 out]
    n215 = local write "Tabla"(w50) -> ()
  }
  n216 = while {
    tunnel: w15 -> [w515]
    tunnel: [w517] -> w24
    tunnel: w11 -> [w520]
    stop <- w521 stop-if-true
    n217 = event shown="[4] \"genera2\": Value Change" {
      selector: w520 -> [_ _ _ _ _ _ _ _ _ _ _]
      dyn-events: _ -> [_ _ _ _ _ _ _ _ _ _ _]
      timeout: _ -> [_ _ _ _ _ _ _ _ _ _ _]
      tunnel: w515 -> [w524 _ w535 w542 w548 w553 w555 w562 w567 w571 w575]
      tunnel: [w527 _ _ w543 w545 w550 w556 w563 w566 w570 w572] -> w518
      tunnel: [_ w528 _ _ _ _ _ _ _ _ _] -> w519
      event "salir": Value Change {
        n218 = event-data() -> ()  [unwired: 1 in, 1 out]
        n219 = call-poly "Enqueue Message.vi"("Message"="Detener_Instrumento", "Message Queue"=w524) -> ("error out"=w522:errorcluster, "dup Message Queue"=w523:refnum<queue>)  [unwired: 8 in]
        n220 = call-poly "Enqueue Message.vi"("error in (no error)"=w522, "Message"="Exit", "Message Queue"=w523) -> ("error out"=w527:errorcluster)  [unwired: 7 in, 1 out]
      }
      event User Event {
        n221 = event-data() -> ("User Event"=w530:string, "Event Data"=w529:variant)  [unwired: 1 in]
        n222 = case shown="\"Exit EHL\"" w530 {
          tunnel: w529 -> [_ w532]
          tunnel: [_ w531] -> w528
          frame Default {
          }
          frame "Exit EHL" {
            # "#evangelio Termina\nla ejecucion del EHL"
            n223 = Variant To Data(type=TRUE, Variant=w532) -> (data=w531:bool)  [unwired: 1 in, 1 out]
          }
        }
      }
      event Panel Close? {
        w534 = TRUE
        n224 = event-data() -> ()  [unwired: 1 in, 1 out]
        n225 = call-poly "Enqueue Message.vi"("Priority Message? (F)"=w534, "Message"="Confirmar Salida", "Message Queue"=w535) -> ()  [unwired: 7 in, 2 out]
        n226 = event-data("Discard?"=w534) -> ()  [unwired: 1 in, 1 out]
      }
      event "generar1": Value Change {
        n227 = event-data() -> ("NewVal"=w541:bool)  [unwired: 1 in]
        n228 = Select(t="iniciarGEN_1", s=w541, f="detenerGEN") -> (s? t:f=w538:string)
        n229 = call-poly "Enqueue Message.vi"("Priority Message? (F)"=TRUE, "Message"=w538, "Message Queue"=w542) -> ("error out"=w543:errorcluster)  [unwired: 7 in, 1 out]
      }
      event "genera2": Value Change {
        n230 = event-data() -> ()  [unwired: 1 in, 1 out]
        n231 = call-poly "Enqueue Message.vi"("Message"="iniciarGEN_burst", "Message Queue"=w548) -> ("error out"=w546:errorcluster)  [unwired: 8 in, 1 out]
        n232 = property on="TablaTempotal" class="Tbl (strict)"(error in=w546, "DisabledEnum"=T6."Enabled" ("Disabled")) -> (error out=w545:errorcluster)  [unwired: 1 in, 1 out]
      }
      event "seguir": Value Change {
        (unwired) T8 {"Estados"=enum."nivelMaxRef", "Data"=variant} ("MessageP08")
        n233 = event-data() -> ()  [unwired: 1 in, 1 out]
        n234 = call-poly "Enqueue Message.vi"("Message"="nivelMaxRef", "Message Queue"=w553) -> ("error out"=w551:errorcluster)  [unwired: 8 in, 1 out]
        n235 = property on="Tab" class="TabCtl (strict)"(error in=w551, "Value"=enum32{"Page 1", "Page 2"}."Page 2" ("Tab")) -> (error out=w550:errorcluster)  [unwired: 1 in, 1 out]
      }
      event "guardarParamLEQ": Value Change {
        (unwired) T8 {"Estados"=enum."nivelMaxRef", "Data"=variant} ("MessageP08")
        n236 = event-data() -> ()  [unwired: 1 in, 1 out]
        n237 = call-poly "Enqueue Message.vi"("Message"="nivelMaxRef", "Message Queue"=w555) -> ("error out"=w556:errorcluster)  [unwired: 8 in, 1 out]
      }
      event Value Change {
        n238 = event-data() -> ()  [unwired: 1 in, 1 out]
        n239 = Divide(x="AjusteAmp", y=T1 1000.0) -> (x/y=w558:T1)
        n240 = call-poly "Enqueue Message.vi"("Priority Message? (F)"=TRUE, "Message Data"=w558, "Message"="EnviarVoltajeGEN", "Message Queue"=w562) -> ("error out"=w563:errorcluster)  [unwired: 6 in, 1 out]
      }
      event "guardar_Vref": Value Change {
        n241 = event-data() -> ()  [unwired: 1 in, 1 out]
        n242 = call-poly "Enqueue Message.vi"("Priority Message? (F)"=TRUE, "Message"="guardaVref", "Message Queue"=w567) -> ("error out"=w566:errorcluster)  [unwired: 7 in, 1 out]
      }
      event "TablaTempotal": Value Change {
        n243 = event-data() -> ("NewVal"=w569:string[][])  [unwired: 1 in]
        n244 = call-poly "Enqueue Message.vi"("Message Data"=w569, "Message"="llenaTablaTemporal", "Message Queue"=w571) -> ("error out"=w570:errorcluster)  [unwired: 7 in, 1 out]
      }
      event "cb_ponderacionTemp": Value Change {
        n245 = event-data() -> ("NewVal"=w573:string)  [unwired: 1 in]
        n246 = call-poly "Enqueue Message.vi"("Message Data"=w573, "Message"="TipoPonderacionTemporal", "Message Queue"=w575) -> ("error out"=w572:errorcluster)  [unwired: 7 in, 1 out]
      }
    }
    n247 = call "Error Handler - Event Handling Loop.vi"("error in (no error)"=w518, "Message Queue"=w515) -> ("dup error in"=w517:errorcluster, "Error?"=w516:bool)  [unwired: 7 in, 1 out]
    n248 = Or(x=w519, y=w516) -> (x .or. y?=w521:bool)
  }
  n249 = call "Inst_CNT90.vi"("All Message Queues in"=w9, "Prueba31 in"=w10) -> ()  [unwired: 9 in, 1 out]
  n250 = call "Inst_DS360.vi"("All Message Queues in"=w9, "Prueba08 in"=w10) -> ()  [unwired: 9 in, 1 out]
  n251 = call "Inst_K2002.vi"("All Message Queues in"=w9, "Prueba31 in"=w10) -> ()  [unwired: 9 in, 1 out]
  n252 = call-dynamic "CleanUp.vi"("Prueba08 in"=w4) -> ("error out"=w1:errorcluster, "Prueba08 out"=→"Prueba08 out":refnum<class "Prueba08.lvclass">)  [unwired: 9 in]
  n253 = Merge Errors(w24, w1, w2) -> (→"error out":errorcluster)
